vi "Histogram Comparison.vi"(8 "error in":errorcluster, 10 "Image 2":path, 11 "Image 1":path) -> (0 "error out":errorcluster, 2 "Histogram Graphs":T1, 3 "Histogram Comparison Score":dbl)   [LabVIEW 2015, in "Histogram Comparison.lvclass"]
uses:
  Histogram Comparison.lvclass
  Image Comparison/Image Comparison.lvclass
  <vilib>/Analysis/NI_AALBase.lvlib
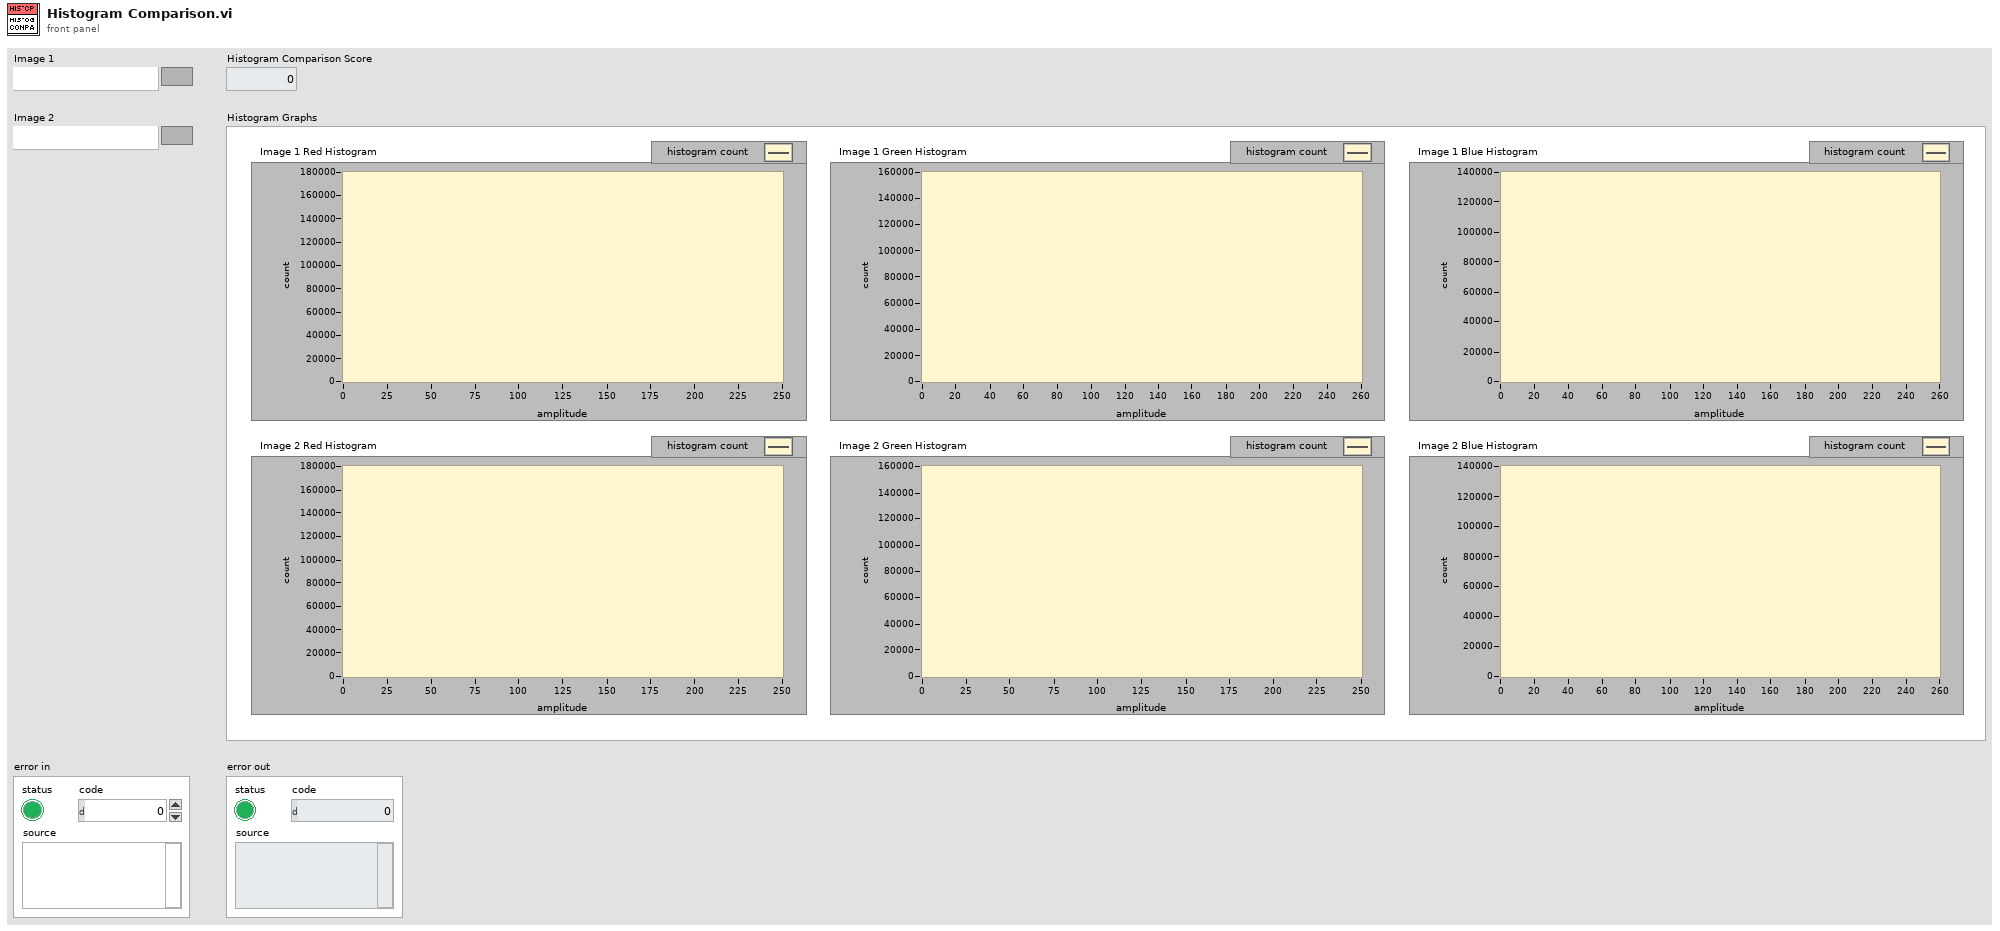
[diagram p1: front panel]
types:
  T1 = cluster{"Image 1 Red Histogram":cluster{"X Values":dbl[], "Histogram: h(x)":i32[]}, "Image 1 Green Histogram":cluster{"X Values":dbl[], "Histogram: h(x)":i32[]}, "Image 1 Blue Histogram":cluster{"X Values":dbl[], "Histogram: h(x)":i32[]}, "Image 2 Red Histogram":cluster{"X Values":dbl[], "Histogram: h(x)":i32[]}, "Image 2 Green Histogram":cluster{"X Values":dbl[], "Histogram: h(x)":i32[]}, "Image 2 Blue Histogram":cluster{"X Values":dbl[], "Histogram: h(x)":i32[]}}
  T2 = typedef "imagedata.ctl" = cluster{"image type":i32, "image depth":i32, "image":u8[], "mask":u8[], "colors":u32[], "Rectangle":cluster{"left":i16, "top":i16, "right":i16, "bottom":i16}}
  T3 = cluster{"X Values":dbl[], "Histogram: h(x)":i32[]}
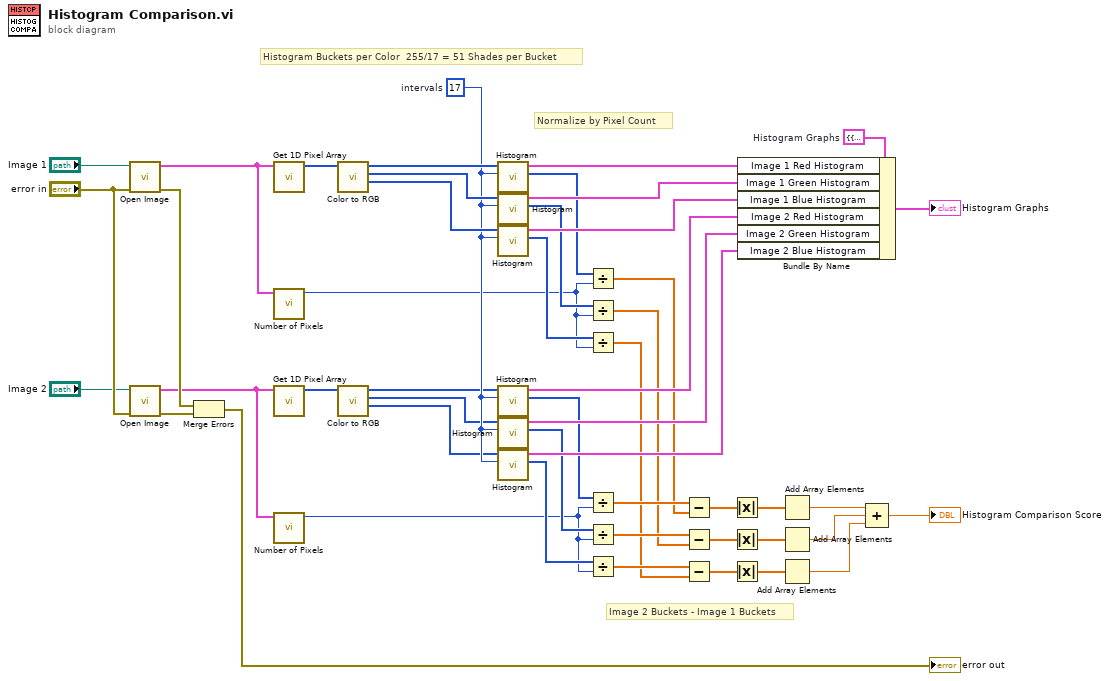
[diagram p0: block diagram]
diagram:
  w41 = T1 {"Image 1 Red Histogram"={"X Values"=[], "Histogram: h(x)"=[]}, "Image 1 Green Histogram"={"X Values"=[], "Histogram: h(x)"=[]}, "Image 1 Blue Histogram"={"X Values"=[], "Histogram: h(x)"=[]}, "Image 2 Red Histogram"={"X Values"=[], "Histogram: h(x)"=[]}, "Image 2 Green Histogram"={"X Values"=[], "Histogram: h(x)"=[]}, "Image 2 Blue Histogram"={"X Values"=[], "Histogram: h(x)"=[]}}  # Histogram Graphs
  w37 = 17  # intervals
  # "Image 2 Buckets - Image 1 Buckets"
  # "Normalize by Pixel Count"
  # "Histogram Buckets per Color  255/17 = 51 Shades per Bucket"
  n1 = call "Open Image.vi"("error in (no error)"="error in", "Image"="Image 1") -> ("error out"=w47:errorcluster, "image data"=w2:T2)  [unwired: 8 in]
  n2 = call "Open Image.vi"("error in (no error)"="error in", "Image"="Image 2") -> ("error out"=w46:errorcluster, "image data"=w4:T2)  [unwired: 8 in]
  n3 = Merge Errors(w47, w46) -> (→"error out":errorcluster)
  n4 = call "Get 1D Pixel Array.vi"("image data"=w2) -> ("1D Pixel Array"=w44:u32[])  [unwired: 10 in]
  n5 = call "Number of Pixels.vi"("image data"=w2) -> ("Number of Pixels"=w1:u64)  [unwired: 10 in]
  n6 = call "Get 1D Pixel Array.vi"("image data"=w4) -> ("1D Pixel Array"=w8:u32[])  [unwired: 10 in]
  n7 = call "Number of Pixels.vi"("image data"=w4) -> ("Number of Pixels"=w3:u64)  [unwired: 10 in]
  n8 = call "Color to RGB.vi"("1D Pixel Array"=w44) -> ("Blue[]"=w38:u8[], "Green[]"=w40:u8[], "Red[]"=w43:u8[])  [unwired: 8 in]
  n9 = call "Color to RGB.vi"("1D Pixel Array"=w8) -> ("Blue[]"=w5:u8[], "Green[]"=w6:u8[], "Red[]"=w7:u8[])  [unwired: 8 in]
  n10 = call <vilib>:"Histogram.vi"("intervals"=w37, "X"=w43) -> ("Histogram: h(x)"=w30:i32[], "Histogram Graph"=w42:T3)  [unwired: 6 in, 2 out]
  n11 = call <vilib>:"Histogram.vi"("intervals"=w37, "X"=w40) -> ("Histogram: h(x)"=w29:i32[], "Histogram Graph"=w39:T3)  [unwired: 6 in, 2 out]
  n12 = call <vilib>:"Histogram.vi"("intervals"=w37, "X"=w38) -> ("Histogram: h(x)"=w28:i32[], "Histogram Graph"=w36:T3)  [unwired: 6 in, 2 out]
  n13 = call <vilib>:"Histogram.vi"("intervals"=w37, "X"=w7) -> ("Histogram: h(x)"=w27:i32[], "Histogram Graph"=w35:T3)  [unwired: 6 in, 2 out]
  n14 = call <vilib>:"Histogram.vi"("intervals"=w37, "X"=w6) -> ("Histogram: h(x)"=w26:i32[], "Histogram Graph"=w34:T3)  [unwired: 6 in, 2 out]
  n15 = call <vilib>:"Histogram.vi"("intervals"=w37, "X"=w5) -> ("Histogram: h(x)"=w25:i32[], "Histogram Graph"=w33:T3)  [unwired: 6 in, 2 out]
  n16 = Divide(x=w30, y=w1) -> (x/y=w23:dbl[])
  n17 = Divide(x=w29, y=w1) -> (x/y=w21:dbl[])
  n18 = Divide(x=w28, y=w1) -> (x/y=w19:dbl[])
  n19 = Divide(x=w27, y=w3) -> (x/y=w24:dbl[])
  n20 = Divide(x=w26, y=w3) -> (x/y=w22:dbl[])
  n21 = Divide(x=w25, y=w3) -> (x/y=w20:dbl[])
  n22 = Subtract(x=w24, y=w23) -> (x-y=w18:dbl[])
  n23 = Subtract(x=w22, y=w21) -> (x-y=w17:dbl[])
  n24 = Subtract(x=w20, y=w19) -> (x-y=w16:dbl[])
  n25 = Absolute Value(x=w18) -> (abs(x)=w15:dbl[])
  n26 = Absolute Value(x=w17) -> (abs(x)=w14:dbl[])
  n27 = Absolute Value(x=w16) -> (abs(x)=w13:dbl[])
  n28 = Bundle By Name(cluster=w41, "Image 1 Red Histogram"=w42, "Image 1 Green Histogram"=w39, "Image 1 Blue Histogram"=w36, "Image 2 Red Histogram"=w35, "Image 2 Green Histogram"=w34, "Image 2 Blue Histogram"=w33) -> (→"Histogram Graphs":T1)
  n29 = Add Array Elements(numeric array=w15) -> (sum=w12:dbl)
  n30 = Add Array Elements(numeric array=w14) -> (sum=w11:dbl)
  n31 = Add Array Elements(numeric array=w13) -> (sum=w10:dbl)
  n32 = Compound Arithmetic op=ADD(w12, w11, w10) -> (→"Histogram Comparison Score":dbl)
